vi "传输内容编码.vi"(11 "输入":T1 {"信息内容" format="%02x"}) -> (3 "输出数组":u8[](array[numeric]) format="%02xH")   [LabVIEW 2016, in "环境动力监测库.lvlib" / "NMEA.lvlib"]
uses:
  NMEA.lvlib
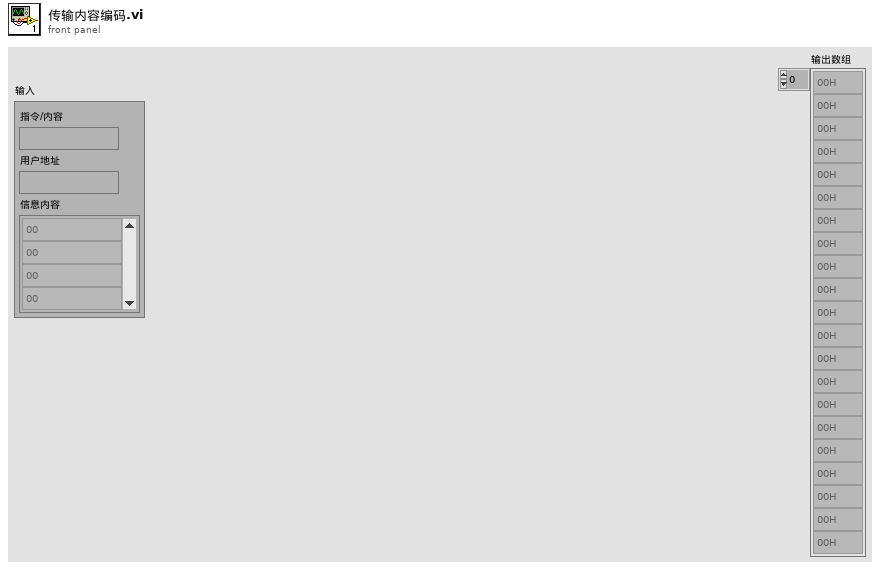
[diagram p1: front panel]
types:
  T1 = cluster{"指令/内容":string, "用户地址":string, "信息内容":u8[]}
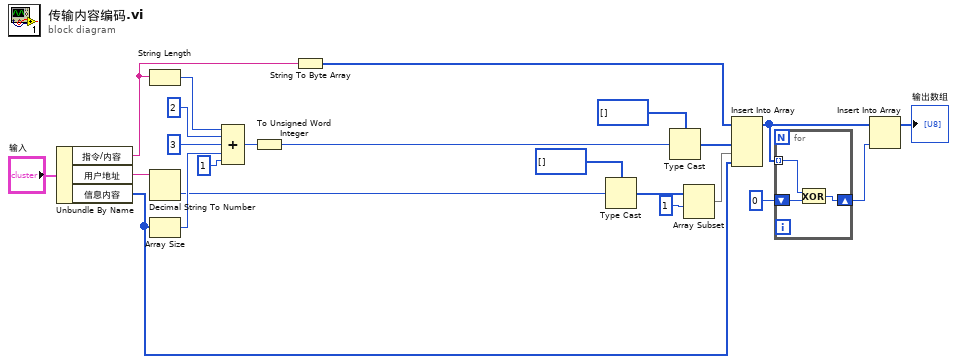
[diagram p0: block diagram]
diagram:
  n1 = Unbundle By Name("输入") -> ("指令/内容"=w17:string, "用户地址"=w3:string, "信息内容"=w13:u8[])
  n2 = String Length(string=w17) -> (length=w16:i32)
  n3 = Decimal String To Number(string=w3) -> (number=w7:i32)  [unwired: 2 in, 1 out]
  n4 = Array Size(array=w13) -> (size(s)=w12:i32)
  n5 = Compound Arithmetic op=ADD(w16, 2 ("y"), 3 ("y"), w12, 1 ("y")) -> (w15:i32)
  n6 = To Unsigned Word Integer(number=w15) -> (unsigned 16bit integer=w21:u16)
  n7 = String To Byte Array(string=w17) -> (unsigned byte array=w22:u8[])
  n8 = Type Cast(type=u8[] [], x=w7) -> (*(type *) &x=w5:u8[])
  n9 = Type Cast(type=u8[] [], x=w21) -> (*(type *) &x=w19:u8[])
  n10 = Array Subset(array=w5, index=1 ("索引")) -> (w2:u8[])  [unwired: 1 in]
  n11 = Insert Into Array(array=w22, new element #1=w19, new element #2=w2, new element #3=w13) -> (w10:u8[])  [unwired: 1 in]
  n12 = for {
    tunnel: w10 -> [w26] mode=indexing
    shift-right: [w25] -> w9
    shift-left: u8 0 -> [w24]
    n13 = Exclusive Or(1:w24, 2:w26) -> (0:w25:u8)
  }
  n14 = Insert Into Array(array=w10, new element=w9) -> (→"输出数组":u8[])  [unwired: 1 in]
